vi "MT Generate QAM System Parameters(map).vi"(0 "samples per symbol (16)":i32=16, 5 "symbol values":i32[][](array[numeric]), 11 "error in (no error)":errorcluster) -> (6 "QAM system parameters":T1 {"symbol map" format="%.3f"}, 8 "bits per symbol":i32, 15 "error out":errorcluster)   [LabVIEW 2020, in "niDMT.lvlib"]
doc: "This polymorphic instance calculates parameters for use with either the MT Modulate QAM VI or the MT Demodulate QAM VI. It accepts an input array of <B>symbol values</B> that explicitly specifies the positions of the symbol map."
uses:
  <vilib>/addons/Modulation/niDMT.lvlib
  <vilib>/addons/Modulation/Digital/Support/Controls/QAM System Parameters.ctl
  <vilib>/addons/Modulation/niAMT.lvlib
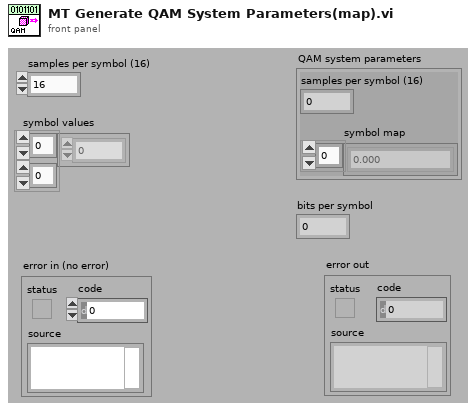
[diagram p1: front panel]
types:
  T1 = cluster{"samples per symbol (16)":i32, "symbol map":cdb[]}
  T2 = typedef "niDMT.lvlib/QAM System Parameters.ctl" = cluster{"samples per symbol (16)":i32, "symbol map":cdb[]}
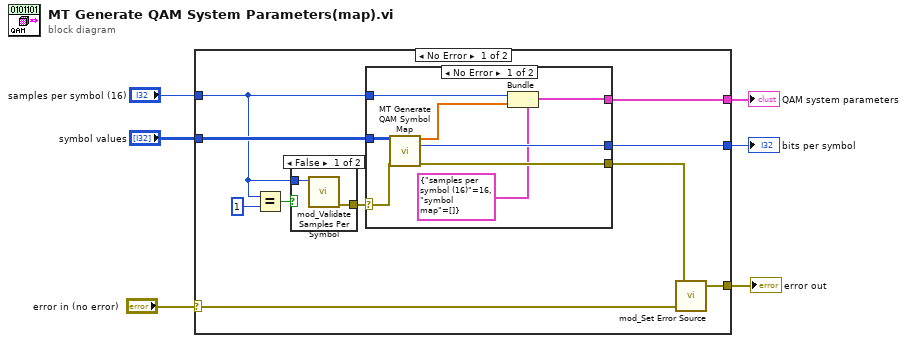
[diagram p0: block diagram]
diagram:
  n1 = case shown="No Error" "error in (no error)" {
    selector: "error in (no error)" -> [w14 w28]
    tunnel: "samples per symbol (16)" -> [w9 _]
    tunnel: [w16 _] -> w5
    tunnel: "symbol values" -> [w11 _]
    tunnel: [w15 _] -> w3
    tunnel: [w13 w28] -> w2
    frame No Error {
      n2 = Equal?(x=w9, y=1) -> (x = y?=w7:bool)
      n3 = case shown="False" w7 {
        tunnel: w9 -> [w18 _]
        tunnel: [w17 _] -> w10
        frame False {
          n4 = call <vilib>:"mod_Validate Samples Per Symbol.vi"("Samples Per Symbol"=w18) -> ("error out"=w17:errorcluster)  [unwired: 10 out]
        }
        frame True {
        }
      }
      n5 = case shown="No Error" w10 {
        selector: w10 -> [w20 w27]
        tunnel: [w26 _] -> w16
        tunnel: [w24 _] -> w15
        tunnel: [w23 w27] -> w12
        tunnel: w11 -> [w22 _]
        tunnel: w9 -> [w21 _]
        frame No Error {
          n6 = call <vilib>:"MT Generate QAM Symbol Map.vi"("symbol values"=w22, "error in (no error)"=w20) -> ("symbol map"=w25:cdb[], "bits per symbol"=w24:i32, "error out"=w23:errorcluster)  [unwired: 11 out]
          n7 = Bundle(cluster=T2 {"samples per symbol (16)"=16, "symbol map"=[]} ("QAM system parameters"), "samples per symbol (16)"=w21, "symbol map"=w25) -> (w26:T2)
        }
        frame Error {
        }
      }
      n8 = call <vilib>:"mod_Set Error Source.vi"("initial error in (no error)"=w14, "final error in (no error)"=w12) -> ("error out"=w13:errorcluster)  [unwired: 3 out]
    }
    frame Error {
    }
  }
  "QAM system parameters" <- w5
  "bits per symbol" <- w3
  "error out" <- w2
